vi "总磷氨氮启动参数对话框.vi"() -> (2 "确认":bool, 3 "元素":cluster{"命令":string, "data":variant})   [LabVIEW 2016, in "氨氮总磷.lvlib"]
panel:
  in  "站号":u16(ring)=1 items=["总磷"=1, "氨氮"=3]
  in  "取消":bool
  in  "确定":bool
  in  "测量间隔":u16
  in  "模式设置":T1(ring)
  out "系统时间":timestamp format="%<%x %X>T"
  out "仪器时间":timestamp format="%<%x %X>T"
  in  "量程切换":enum32{"H", "L", "AUTO"}(radio)=enum."AUTO"
  in  "控制命令":T2(ring)
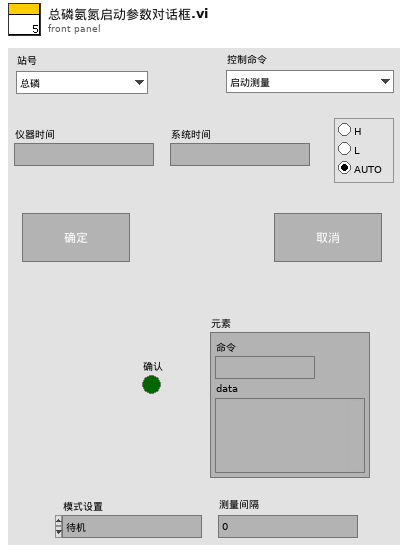
[diagram p1: front panel]
types:
  T1 = enum16{"待机", "连续模式", "周期模式", "定点模式", "受控模式", "手动模式"}
  T2 = enum16{"启动测量", "标样核查", "零点核查", "跨度核查", "空白测试", "平行样测试", "加标回收", "空白校准", "标样校准", "初始化（清洗）", "停止测试", "仪器重启", "校时", "模式设置", "测量间隔设置"}
  T3 = cluster{"站号":u16, "量程切换":enum32{"H", "L", "AUTO"}, "控制命令":enum16{"启动测量", "标样核查", "零点核查", "跨度核查", "空白测试", "平行样测试", "加标回收", "空白校准", "标样校准", "初始化（清洗）", "停止测试", "仪器重启", "校时", "模式设置", "测量间隔设置", "盲样测试"}, "模式设置":enum16{"待机", "连续模式", "周期模式", "定点模式", "受控模式", "手动模式"}, "测量间隔":u16}
  T4 = cluster{"系统时间":timestamp, "工作状态":enum16{"空闲", "水样测试", "标样核查", "零点核查", "跨度核查", "空白测试", "平行样测试", "加标回收", "空白校准", "标样校准", "初始化（清洗）"}, "测量模式":enum16{"待机", "连续模式", "周期模式", "定点模式", "受控模式", "手动模式"}, "告警代码":enum16{"无告警", "缺试剂告警", "缺水样告警", "缺蒸馏水告警", "缺标液告警", "仪表漏液告警", "标定异常告警", "超量程告警", "加热异常", "低试剂预警", "超上限告警", "超下限告警", "仪表内部其他异常", "滴定异常告警", "电极异常告警", "量程切换告警", "参数设置告警", "PH电极电位异常", "电导率电极异常", "浊度光度异常", "溶解氧电极异常", "溶解氧光强异常", "温度异常告警", "PH异常告警", "溶解氧异常告警", "电导率异常告警", "浊度异常告警", "叶绿素异常告警", "藻密度异常告警", "蓝绿藻异常告警", "ORP异常告警", "氨氮异常告警", "清洁刷异常告警", "SD卡异常告警", "蓝牙异常告警", "Wifi异常告警", "流程异常告警"}, "故障代码":enum16{"无故障", "电机故障", "温度故障", "通讯故障", "滴定故障"}, "日志代码":u16, "软件版本":u16, "F0":sgl, "F1":sgl, "F2":sgl, "F3":sgl, "T":sgl, "H":sgl, "id":u16, "flowid":u16, "量程":u16, "总磷控温温度1":sgl, "营养盐控温温度2":sgl, "ADC":sgl}
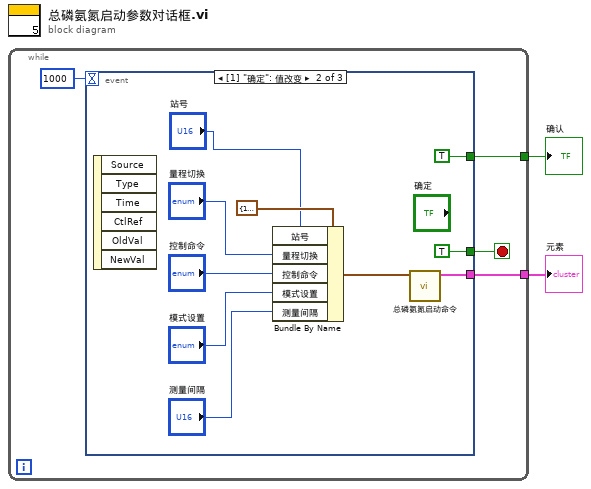
[diagram p0: block diagram]
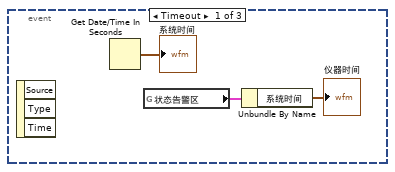
[diagram p2: hidden frame]
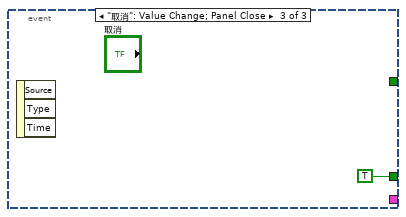
[diagram p3: hidden frame]
diagram:
  n1 = while {
    tunnel: [w4] -> w2
    tunnel: [w3] -> w1
    stop <- w6 stop-if-true
    n2 = event shown="[1] \"确定\": 值改变" {
      selector: _ -> [_ _ _]
      dyn-events: _ -> [_ _ _]
      timeout: 1000 -> [_ _ _]
      tunnel: [_ TRUE TRUE] -> w6
      tunnel: [_ TRUE _] -> w4
      tunnel: [_ w17 _] -> w3
      event Timeout {
        n3 = event-data() -> ()  [unwired: 1 in, 3 out]
        n4 = Get Date/Time In Seconds() -> (seconds since 1Jan1904=→"系统时间":timestamp)
        n5 = global read "VAR总磷氨氮全局变量.vi" "状态告警区"() -> (w7:T4)
        n6 = Unbundle By Name(w7) -> ("系统时间"=→"仪器时间":timestamp)
      }
      event "确定": Value Change {
        n7 = event-data() -> ()  [unwired: 1 in, 6 out]
        n8 = Bundle By Name(cluster=T3 {"站号"=1, "量程切换"=enum."AUTO", "控制命令"=enum."启动测量", "模式设置"=enum."待机", "测量间隔"=0} ("参数"), "站号"="站号", "量程切换"="量程切换", "控制命令"="控制命令", "模式设置"="模式设置", "测量间隔"="测量间隔") -> (w15:T3)
        n9 = call "总磷氨氮启动命令.vi"("参数"=w15) -> ("启动命令"=w17:cluster{"命令":string, "data":variant})  [unwired: 10 in]
      }
      event "取消": Value Change; Panel Close {
        n10 = event-data() -> ()  [unwired: 1 in, 3 out]
      }
    }
  }
  "元素" <- w1
  "确认" <- w2
